vi "E02.vi"() -> ()   [LabVIEW 2020]
panel:
  in  "Botón de paro":bool
  out "n!":i32
  in  "n":i32
  # "Calculadora de factorial"
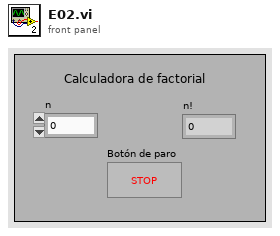
[diagram p1: front panel]
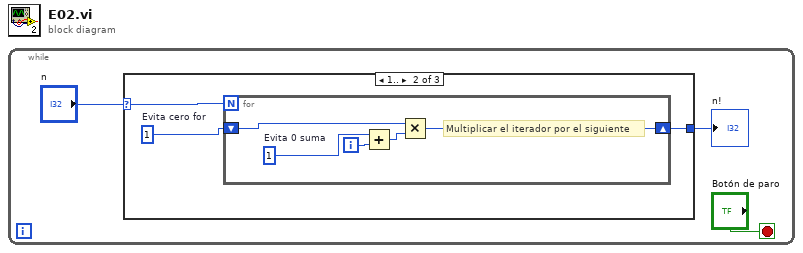
[diagram p0: block diagram]
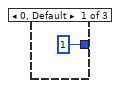
[diagram p2: hidden frame]
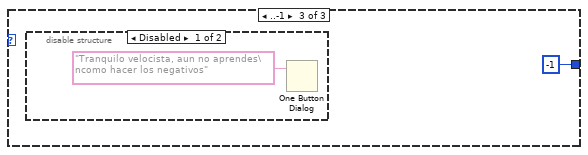
[diagram p3: hidden frame]
diagram:
  n1 = while {
    stop <- "Botón de paro" stop-if-true
    n2 = case shown="1.." "n" {
      selector: "n" -> [_ w7 _]
      tunnel: [1 w5 -1] -> w3
      frame 0, Default {
      }
      frame 1.. {
        w6 = 1  # Evita cero for
        n3 = for {
          N: w7 -> [_]
          shift-right: [w11] -> w5
          shift-left: w6 -> [w12]
          i -> [w10]
          w8 = 1  # Evita 0 suma
          # "Multiplicar el iterador por el siguiente"
          n4 = Add(x=w8, y=w10) -> (x+y=w9:i32)
          n5 = Multiply(x=w12, y=w9) -> (x*y=w11:i32)
        }
      }
      frame ..-1 {
        n6 = disable-structure shown="Disabled" {
          frame Disabled {
            n7 = One Button Dialog(message="Tranquilo velocista, aun no aprendes\ncomo hacer los negativos") -> ()  [unwired: 1 in, 1 out]
          }
          frame Enabled {
          }
        }
      }
    }
    "n!" <- w3
  }
